vi "createFreezeSensorValuesFrame.vi"(0 "HardPointActuator in":refnum<class "HPILC.lvclass">, 5 "WaitForTrigger":bool, 7 "TriggerIRQ":bool, 9 "BroadcastCounter":u8, 11 "error in (no error)":errorcluster) -> (4 "HardPointActuator out":refnum<class "HPILC.lvclass">, 6 "Frame":T1 {"Data" format="%02x"}, 15 "error out":errorcluster)   [LabVIEW 2016, in "RTHPILC.lvlib" / "HPILC.lvclass"]
uses:
  HPILC.lvclass
  Common_RT_Modbus/DataTypes/Frame.ctl
  Common_RT_Modbus/DynamicFrameBuilder/DynamicFrameBuilder.lvclass
  HPILC.lvclass/HPILC.ctl
  Common_RT_Modbus/RTModbus.lvlib
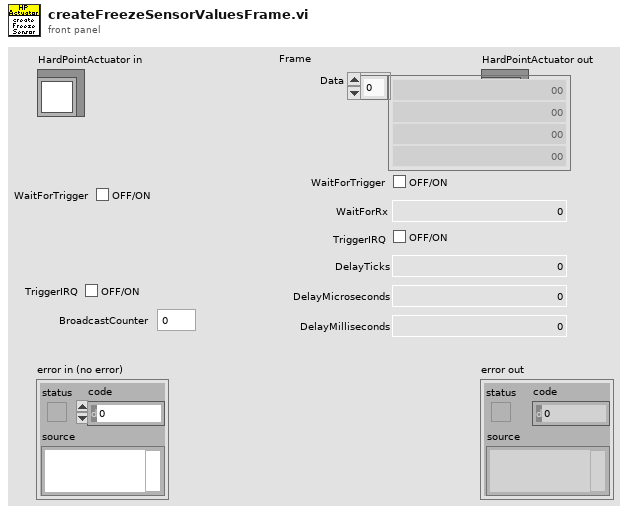
[diagram p1: front panel]
types:
  T1 = typedef "RTModbus.lvlib/Frame.ctl" = cluster{"Data":u8[], "WaitForTrigger":bool, "WaitForRx":u16, "TriggerIRQ":bool, "DelayTicks":u16, "DelayMicroseconds":u16, "DelayMilliseconds":u16}
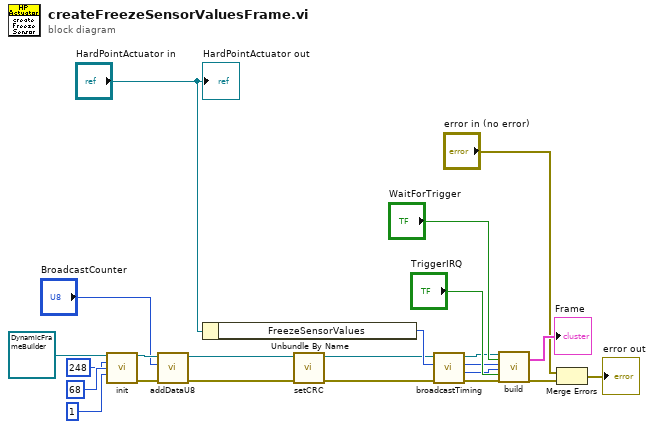
[diagram p0: block diagram]
diagram:
  n1 = call "init.vi"("DynamicFrameBuilder in"=refnum<class "DynamicFrameBuilder.lvclass"> refnum ("RTModbus.lvlib:DynamicFrameBuilder.lvclass"), "Address"=u8 248, "Function"=u8 68, "DataSize"=1) -> ("DynamicFrameBuilder out"=w13:refnum<class "DynamicFrameBuilder.lvclass">, "error out"=w11:errorcluster)  [unwired: 10 in]
  n2 = call "addDataU8.vi"("error in (no error)"=w11, "Data"="BroadcastCounter", "DynamicFrameBuilder in"=w13) -> ("error out"=w10:errorcluster, "DynamicFrameBuilder out"=w9:refnum<class "DynamicFrameBuilder.lvclass">)  [unwired: 7 in]
  n3 = Unbundle By Name("HardPointActuator in") -> ("FreezeSensorValues"=w7:u32)
  n4 = call "setCRC.vi"("error in (no error)"=w10, "DynamicFrameBuilder in"=w9) -> ("error out"=w5:errorcluster, "DynamicFrameBuilder out"=w6:refnum<class "DynamicFrameBuilder.lvclass">)  [unwired: 8 in]
  n5 = call "broadcastTiming.vi"("error in (no error)"=w5, "Latency in"=w7, "DynamicFrameBuilder in"=w6) -> ("error out"=w3:errorcluster, "WaitForRxTimeout"=w1:u16, "Latency out"=w2:u32, "DynamicFrameBuilder out"=w4:refnum<class "DynamicFrameBuilder.lvclass">)  [unwired: 5 in]
  n6 = call "build.vi"("DynamicFrameBuilder in"=w4, "WaitForTrigger"="WaitForTrigger", "Latency"=w2, "WaitForRxTimeout"=w1, "TriggerIRQ"="TriggerIRQ", "error in (no error)"=w3) -> ("Frame"=→"Frame":T1, "error out"=w19:errorcluster)  [unwired: 11 in, 1 out]
  n7 = Merge Errors("error in (no error)", w19) -> (→"error out":errorcluster)
  "HardPointActuator out" <- "HardPointActuator in"
